vi "Motion Move Relative.vi"(8 "error in (no error)":errorcluster, 10 "Decel?":bool, 11 "Distance":i32) -> (0 "error out":errorcluster)   [LabVIEW 2015, in "Tool Interface.lvlib"]
uses:
  Tool Interface.lvlib
  Tool Typedefs/_Move(R) Cmd Params Cluster--typedef.ctl
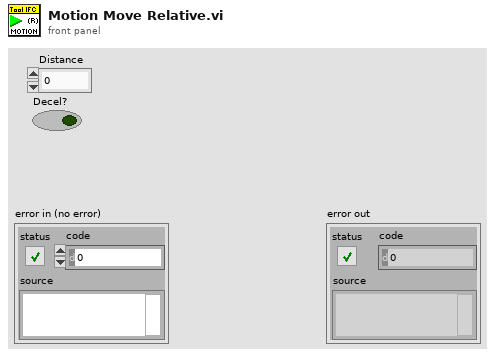
[diagram p1: front panel]
types:
  T1 = typedef "_Move(R) Cmd Params Cluster--typedef.ctl" = cluster{"Distance":i32, "Decel?":bool}
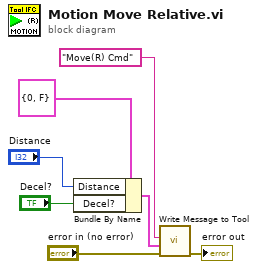
[diagram p0: block diagram]
diagram:
  n1 = Bundle By Name(cluster=T1 {"Distance"=0, "Decel?"=FALSE} ("_Move(R) Cmd Params Cluster--typedef"), "Distance"="Distance", "Decel?"="Decel?") -> (w4:T1)
  n2 = call "Write Message to Tool.vi"("error in (no error)"="error in (no error)", "Message Data"=w4, "Message"="Move(R) Cmd") -> ("error out"=→"error out":errorcluster)  [unwired: 8 in]
